vi "Setup.vi"() -> ()   [LabVIEW 2021, in "Main.lvlib"]
doc: "This VI is used to SetUP the signal properties. \n1.Start SetUP to view the signal\n2. Save Values to save the values that you pick to signal_values FGV\n3. Stop SetUP to stop the SetUP\n5. Exit SetUp"
uses:
  Main.lvlib
  Tipski Definicii/Setup_sostojbi.ctl
  Tipski Definicii/Signal Values.ctl
  Tipski Definicii/Unit.ctl
  Polymorphic/Init_SetUP.vi
  Polymorphic/DeQ_SetUP_QMH.vi
  Polymorphic/Enq_SetUP_QMH.vi
  Polymorphic/Release_SetUP.vi
  Signal/Signal.lvlib
  <vilib>/measure/NI_MABase.lvlib
  subVIS/Main_Programs_SubVIs.lvlib
  Polymorphic/Queues.lvlib
panel:
  in  "Stop SetUP":bool
  in  "Waveform":T1(ring)
  in  "Phase":dbl
  in  "Offset":dbl
  in  "Hz Value":dbl=10000.0 min=-10000.0 max=10000.0 step=0.001 format="%#.3f"
  in  "Amplitude":dbl min=-10.0 max=10.0 step=0.001 format="%#.3f"
  in  "Exit Setup":bool
  in  "Save Values":bool
  in  "Start Setup":bool
  out "Signal":waveform(dbl)(graph)
  # "For DC signal the waveform needs to be square. If you want to pick other waveform first change the f F"
  # "Waveform graph tools"
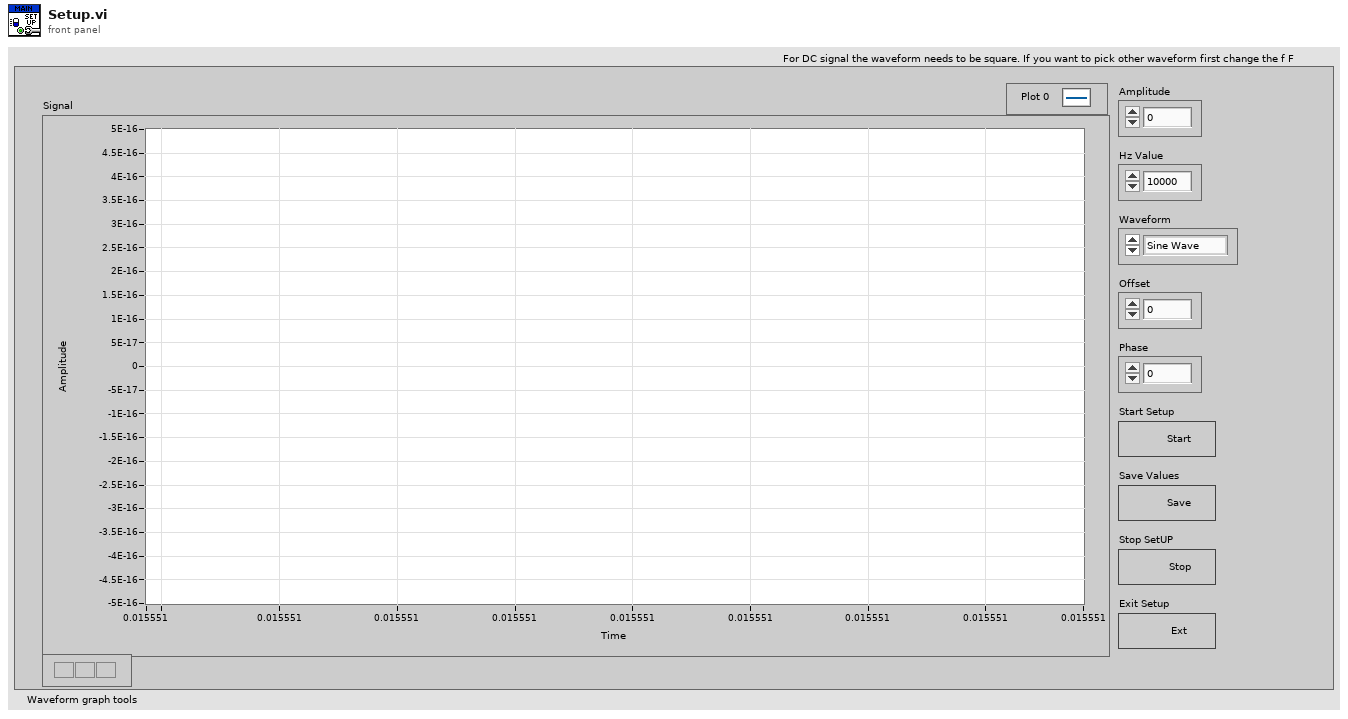
[diagram p1: front panel]
types:
  T1 = enum16{"Sine Wave", "Triangle Wave", "Square Wave", "Sawtooth Wave"}
  T2 = cluster{"Main Queue":refnum<queue>, "ER Refnum":refnum<event-registration>, "User Event":refnum<user-event>}
  T3 = typedef "SetUP_program_queues.ctl" = cluster{"Main Queue":refnum<queue>, "ER Refnum":refnum<event-registration>, "User Event":refnum<user-event>}
  T4 = typedef "Signal Values.ctl" = enum16{"Init", "Add V/A string", "Add Hz string", "Get Strings and Values", "Reset", "Add Offset", "Add Waveform", "Add Phase"}
  T5 = typedef "Setup_sostojbi.ctl" = enum16{"Init", "Generate Message ", "Setup", "End"}
  T6 = enum32{"Invalid", "Standard", "Closed", "Hidden", "Minimized", "Maximized"}
  T7 = cluster{"Amp String":string, "Amp Value":dbl, "Hz Value Out":dbl, "Waveform Out":enum16{"Sine Wave", "Triangle Wave", "Square Wave", "Sawtooth Wave"}, "Offset Out":dbl, "Phase Out":dbl, "Signal String":string, "Signal":waveform(dbl)}
  T8 = typedef "Unit.ctl" = enum16{"Init", "Add", "Read"}
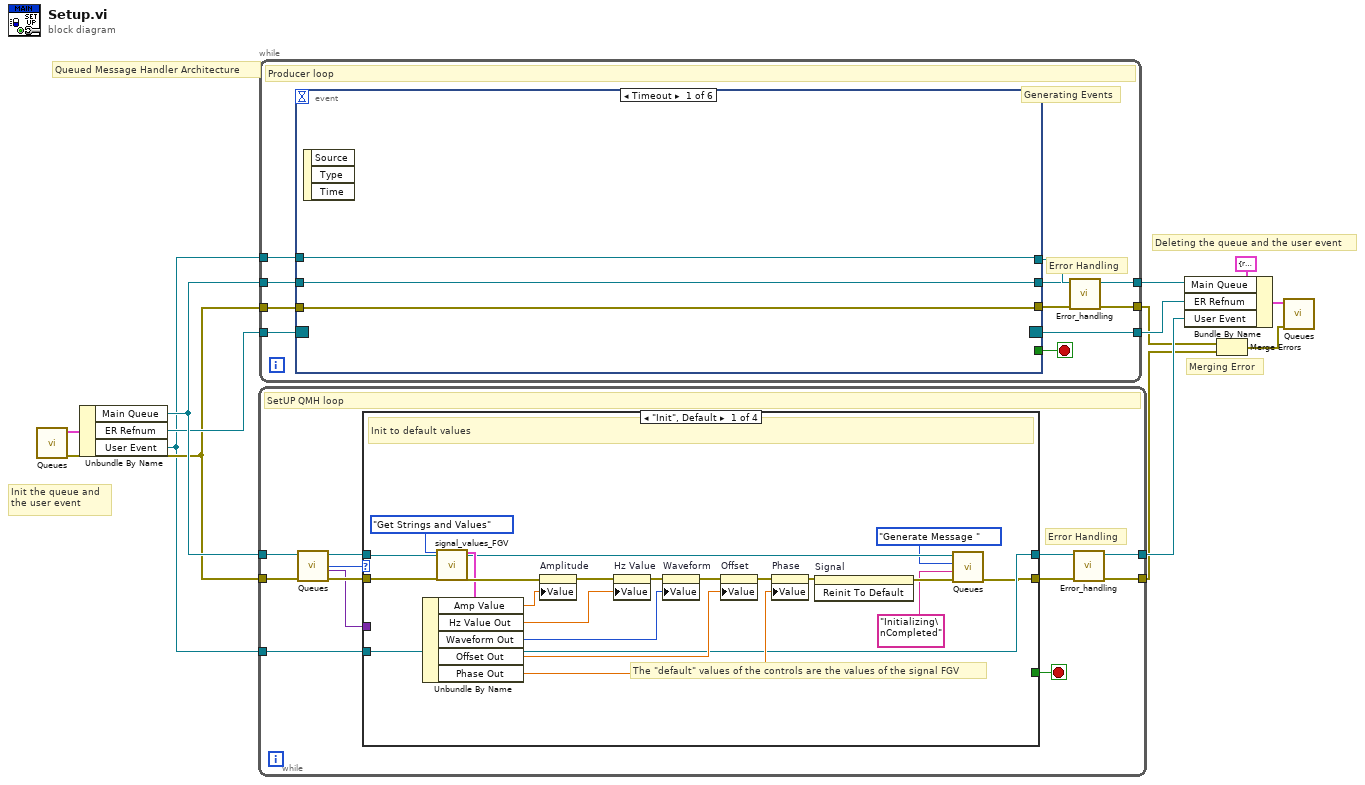
[diagram p0: block diagram]
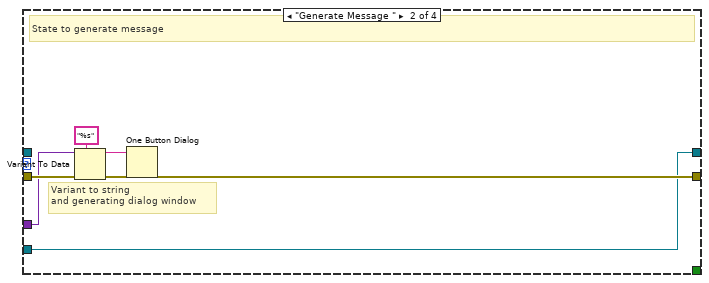
[diagram p2: hidden frame]
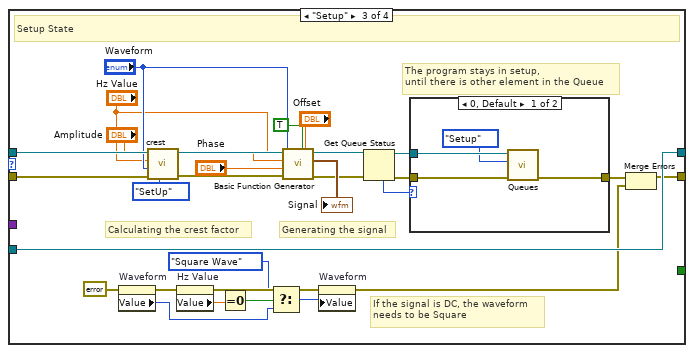
[diagram p3: hidden frame]
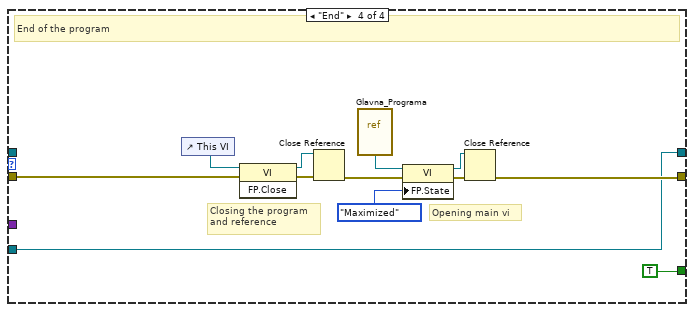
[diagram p5: hidden frame]
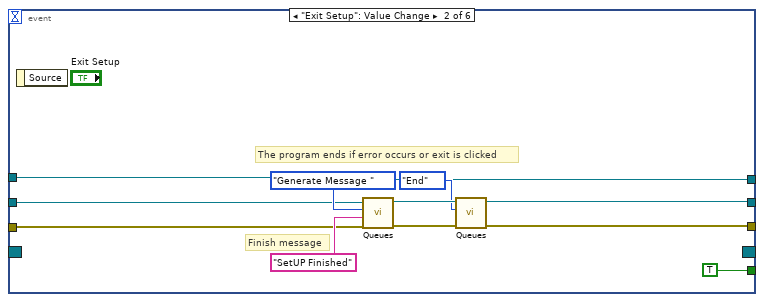
[diagram p6: hidden frame]
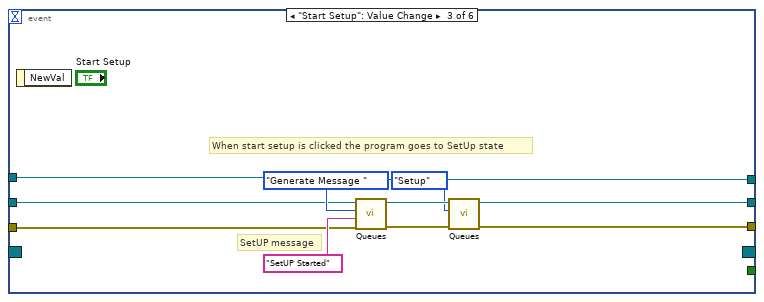
[diagram p7: hidden frame]
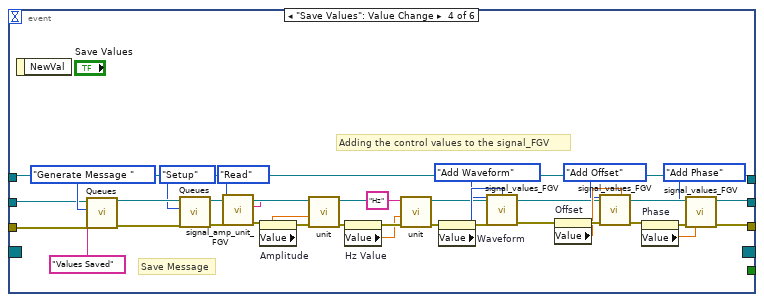
[diagram p8: hidden frame]
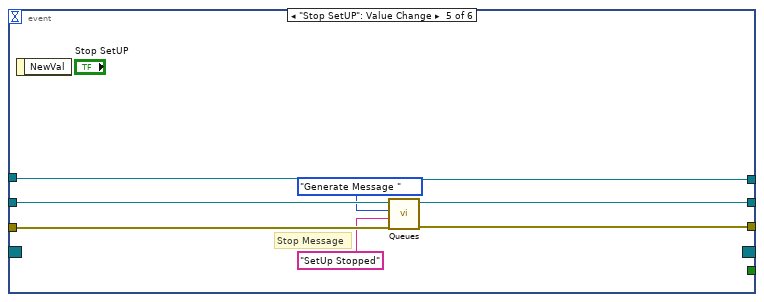
[diagram p9: hidden frame]
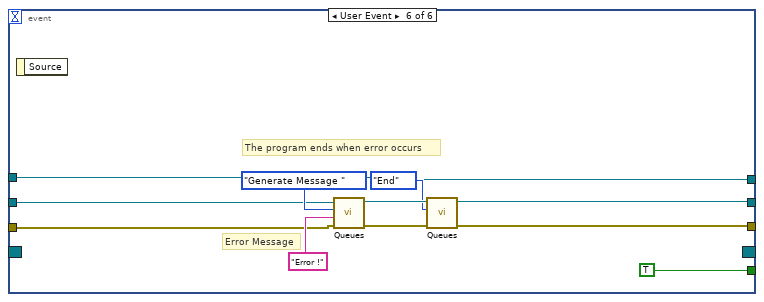
[diagram p10: hidden frame]
diagram:
  # "Merging Error"
  # "Deleting the queue and the user event"
  # "Init the queue and \nthe user event"
  # "Queued Message Handler Architecture"
  n1 = call-poly "Queues.vi"() -> ("Error Out"=w11:errorcluster, "Queue Cluster"=w10:T3)  [unwired: 10 in]
  n2 = Unbundle By Name(w10) -> ("Main Queue"=w13:refnum<queue>, "ER Refnum"=w12:refnum<event-registration>, "User Event"=w9:refnum<user-event>)
  n3 = while {
    tunnel: w13 -> [w18]
    tunnel: [w22] -> w5
    tunnel: w11 -> [w17]
    tunnel: [w24] -> w3
    tunnel: w9 -> [w21]
    stop <- w25 stop-if-true
    # "Error Handling"
    # "SetUP QMH loop"
    n4 = call-poly "Queues.vi"("Error In"=w17, "Queue In"=w18) -> ("Error Out"=w16:errorcluster, "Message"=w14:variant, "Instruction"=w15:T5, "Queue Out"=w19:refnum<queue>)  [unwired: 6 in]
    n5 = case shown="\"Init\", Default" w15 {
      tunnel: w19 -> [w30 _ w71 _]
      tunnel: [w31 w47 w56 w86] -> w23
      tunnel: [_ _ _ TRUE] -> w25
      tunnel: w16 -> [w39 w51 w68 w94]
      tunnel: w14 -> [_ w50 _ _]
      tunnel: w21 -> [w33 w46 w69 w85]
      tunnel: [w33 w46 w69 w85] -> w20
      frame "Init", Default {
        # "The \"default\" values of the controls are the values of the signal FGV"
        # "Init to default values"
        n6 = call "signal_values_FGV.vi"("Action"=Signal_Values."Get Strings and Values", "Error In"=w39) -> ("Signal"=w38:T7, "Error Out"=w45:errorcluster)  [unwired: 12 in]
        n7 = Unbundle By Name(w38) -> ("Amp Value"=w37:dbl, "Hz Value Out"=w36:dbl, "Waveform Out"=w27:T1, "Offset Out"=w35:dbl, "Phase Out"=w34:dbl)
        n8 = property on="Amplitude" class="DigNum (strict)"(error in=w45, "Value"=w37) -> (error out=w44:errorcluster)  [unwired: 1 in, 1 out]
        n9 = property on="Hz Value" class="DigNum (strict)"(error in=w44, "Value"=w36) -> (error out=w43:errorcluster)  [unwired: 1 in, 1 out]
        n10 = property on="Waveform" class="Enum (strict)"(error in=w43, "Value"=w27) -> (error out=w42:errorcluster)  [unwired: 1 in, 1 out]
        n11 = property on="Offset" class="DigNum (strict)"(error in=w42, "Value"=w35) -> (error out=w41:errorcluster)  [unwired: 1 in, 1 out]
        n12 = property on="Phase" class="DigNum (strict)"(error in=w41, "Value"=w34) -> (error out=w40:errorcluster)  [unwired: 1 in, 1 out]
        n13 = invoke on="Signal" class="WFGraph (strict)" method="Reinit To Default"(error in=w40) -> (error out=w32:errorcluster)  [unwired: 2 in, 2 out]
        n14 = call-poly "Queues.vi"("Error In"=w32, "Message"="Initializing\nCompleted", "Instruction"=Setup_sostojbi."Generate Message ", "Queue Out"=w30) -> ("Error Out"=w31:errorcluster)  [unwired: 6 in, 1 out]
      }
      frame "Generate Message " {
        # "Variant to string\nand generating dialog window"
        # "State to generate message"
        n15 = Variant To Data(error in=w51, type="%s", Variant=w50) -> (data=w48:string, error out=w47:errorcluster)
        n16 = One Button Dialog(message=w48) -> ()  [unwired: 1 in, 1 out]
      }
      frame "Setup" {
        # "Calculating the crest factor"
        # "If the signal is DC, the waveform\nneeds to be Square"
        # "The program stays in setup,\nuntil there is other element in the Queue"
        # "Generating the signal"
        # "Setup State"
        n17 = property on="Waveform" class="Enum (strict)"(error in=errorcluster {"status"=FALSE, "code"=0, "source"=""} ("error in (no error)")) -> (error out=w60:errorcluster, "Value"=w59:T1)  [unwired: 1 in, 1 out]
        n18 = call "crest.vi"("Set / Unit?"=enum16{"Unit", "SetUp"}."SetUp", "Error In"=w68, "SetUP W"="Waveform", "SetUP F"="Hz Value", "RMS"="Amplitude") -> ("Error Out"=w67:errorcluster, "Max"=w65:dbl)  [unwired: 5 in]
        n19 = property on="Hz Value" class="DigNum (strict)"(error in=w60) -> (error out=w79:errorcluster, "Value"=w64:dbl)  [unwired: 1 in, 1 out]
        n20 = Equal To 0?(x=w64) -> (x = 0?=w63:bool)
        n21 = Select(t=T1."Square Wave" ("Waveform"), s=w63, f=w59) -> (s? t:f=w58:T1)
        n22 = call <vilib>:"Basic Function Generator.vi"("offset"="Offset", "reset signal"=TRUE, "signal type"="Waveform", "error in (no error)"=w67, "phase"="Phase", "amplitude"=w65, "frequency"="Hz Value") -> ("error out"=w72:errorcluster, "signal out"=→"Signal":waveform(dbl))  [unwired: 2 in, 1 out]
        n23 = property on="Waveform" class="Enum (strict)"(error in=w79, "Value"=w58) -> (error out=w55:errorcluster)  [unwired: 1 in, 1 out]
        n24 = Get Queue Status(queue=w71, error in (no error)=w72) -> (queue out=w74:refnum<queue>, error out=w73:errorcluster, # elements in queue=w75:i32)  [unwired: 1 in, 5 out]
        n25 = case shown="0, Default" w75 {
          tunnel: w74 -> [w82 _]
          tunnel: w73 -> [w83 w84]
          tunnel: [w80 w84] -> w57
          frame 0, Default {
            n26 = call-poly "Queues.vi"("Error In"=w83, "Instruction"=Setup_sostojbi."Setup", "Queue Out"=w82) -> ("Error Out"=w80:errorcluster)  [unwired: 7 in, 1 out]
          }
          frame 1 {
          }
        }
        n27 = Merge Errors(w57, w55) -> (w56:errorcluster)
      }
      frame "End" {
        # "Opening main vi"
        # "Closing the program\nand reference"
        # "End of the program"
        n28 = control-ref of="This VI"() -> (w95:refnum<vi>)
        n29 = invoke class="VI" method="FP.Close"(reference=w95, error in=w94) -> (reference out=w92:refnum<vi>, error out=w93:errorcluster)  [unwired: 1 in, 1 out]
        n30 = Close Reference(reference=w92, error in (no error)=w93) -> (error out=w91:errorcluster)
        n31 = vi-ref "Glavna_Programa.vi"() -> (w90:refnum<vi>)
        n32 = property class="VI"(reference=w90, error in=w91, "FP.State"=T6."Maximized" ("Front Panel Window:State")) -> (reference out=w87:refnum<vi>, error out=w88:errorcluster)
        n33 = Close Reference(reference=w87, error in (no error)=w88) -> (error out=w86:errorcluster)
      }
    }
    n34 = call "Error_handling.vi"("Error In"=w23, "User Event in"=w20) -> ("Error Out"=w24:errorcluster, "User Event out"=w22:refnum<user-event>)  [unwired: 8 in]
  }
  n35 = while {
    tunnel: w11 -> [w105]
    tunnel: w13 -> [w106]
    tunnel: w12 -> [w104]
    tunnel: [w103] -> w6
    tunnel: w9 -> [w101]
    tunnel: [w99] -> w7
    tunnel: [w98] -> w4
    stop <- w97 stop-if-true
    # "Error Handling"
    # "Generating Events"
    # "Producer loop"
    n36 = event shown="[0] Timeout" {
      selector: w104 -> [_ _ _ _ _ _]
      dyn-events: [_ _ _ _ _ _] -> w103
      timeout: _ -> [_ _ _ _ _ _]
      tunnel: w106 -> [w109 w113 w124 w143 w166 w173]
      tunnel: [w109 w112 w121 w139 w167 w172] -> w99
      tunnel: w105 -> [w108 w114 w125 w144 w169 w174]
      tunnel: [w108 w111 w122 w147 w168 w171] -> w102
      tunnel: [_ TRUE _ _ _ TRUE] -> w97
      tunnel: w101 -> [w107 w110 w123 w142 w163 w170]
      tunnel: [w107 w110 w123 w142 w163 w170] -> w100
      event Timeout {
        n37 = event-data() -> ()  [unwired: 1 in, 3 out]
      }
      event "Exit Setup": Value Change {
        # "Finish message"
        # "The program ends if error occurs or exit is clicked"
        n38 = event-data() -> ()  [unwired: 1 in, 1 out]
        n39 = call-poly "Queues.vi"("Error In"=w114, "Message"="SetUP Finished", "Instruction"=Setup_sostojbi."Generate Message ", "Queue Out"=w113) -> ("Error Out"=w118:errorcluster, "Queue Out"=w119:refnum<queue>)  [unwired: 6 in]
        n40 = call-poly "Queues.vi"("Error In"=w118, "Instruction"=Setup_sostojbi."End", "Queue Out"=w119) -> ("Error Out"=w111:errorcluster, "Queue Out"=w112:refnum<queue>)  [unwired: 7 in]
      }
      event "Start Setup": Value Change {
        # "SetUP message"
        # "When start setup is clicked the program goes to SetUp state"
        n41 = event-data() -> ()  [unwired: 1 in, 1 out]
        n42 = call-poly "Queues.vi"("Error In"=w125, "Message"="SetUP Started", "Instruction"=Setup_sostojbi."Generate Message ", "Queue Out"=w124) -> ("Error Out"=w129:errorcluster, "Queue Out"=w130:refnum<queue>)  [unwired: 6 in]
        n43 = call-poly "Queues.vi"("Error In"=w129, "Instruction"=Setup_sostojbi."Setup", "Queue Out"=w130) -> ("Error Out"=w122:errorcluster, "Queue Out"=w121:refnum<queue>)  [unwired: 7 in]
      }
      event "Save Values": Value Change {
        # "Save Message"
        # "Adding the control values to the signal_FGV"
        n44 = event-data() -> ()  [unwired: 1 in, 1 out]
        n45 = call-poly "Queues.vi"("Error In"=w144, "Message"="Values Saved", "Instruction"=Setup_sostojbi."Generate Message ", "Queue Out"=w143) -> ("Error Out"=w141:errorcluster, "Queue Out"=w140:refnum<queue>)  [unwired: 6 in]
        n46 = call-poly "Queues.vi"("Error In"=w141, "Instruction"=Setup_sostojbi."Setup", "Queue Out"=w140) -> ("Error Out"=w134:errorcluster, "Queue Out"=w139:refnum<queue>)  [unwired: 7 in]
        n47 = call "signal_amp_unit_FGV.vi"("Error In"=w134, "Action"=Unit."Read") -> ("Error Out"=w133:errorcluster, "Base"=w131:string)  [unwired: 7 in, 1 out]
        n48 = property on="Amplitude" class="DigNum (strict)"(error in=w133) -> (error out=w162:errorcluster, "Value"=w161:dbl)  [unwired: 1 in, 1 out]
        n49 = call "unit.vi"("Error In"=w162, "Signal Amp"=w161, "Unit"=w131) -> ("Error Out"=w160:errorcluster)  [unwired: 8 in]
        n50 = property on="Hz Value" class="DigNum (strict)"(error in=w160) -> (error out=w159:errorcluster, "Value"=w158:dbl)  [unwired: 1 in, 1 out]
        n51 = call "unit.vi"("Error In"=w159, "Signal Amp"=w158, "Unit"="Hz") -> ("Error Out"=w156:errorcluster)  [unwired: 8 in]
        n52 = property on="Waveform" class="Enum (strict)"(error in=w156) -> (error out=w154:errorcluster, "Value"=w155:T1)  [unwired: 1 in, 1 out]
        n53 = call "signal_values_FGV.vi"("Action"=Signal_Values."Add Waveform", "Waveform"=w155, "Error In"=w154) -> ("Error Out"=w153:errorcluster)  [unwired: 11 in, 1 out]
        n54 = property on="Offset" class="DigNum (strict)"(error in=w153) -> (error out=w152:errorcluster, "Value"=w151:dbl)  [unwired: 1 in, 1 out]
        n55 = call "signal_values_FGV.vi"("Action"=Signal_Values."Add Offset", "Offset"=w151, "Error In"=w152) -> ("Error Out"=w150:errorcluster)  [unwired: 11 in, 1 out]
        n56 = property on="Phase" class="DigNum (strict)"(error in=w150) -> (error out=w149:errorcluster, "Value"=w148:dbl)  [unwired: 1 in, 1 out]
        n57 = call "signal_values_FGV.vi"("Action"=Signal_Values."Add Phase", "Error In"=w149, "Phase"=w148) -> ("Error Out"=w147:errorcluster)  [unwired: 11 in, 1 out]
      }
      event "Stop SetUP": Value Change {
        # "Stop Message"
        n58 = event-data() -> ()  [unwired: 1 in, 1 out]
        n59 = call-poly "Queues.vi"("Error In"=w169, "Message"="SetUp Stopped", "Instruction"=Setup_sostojbi."Generate Message ", "Queue Out"=w166) -> ("Error Out"=w168:errorcluster, "Queue Out"=w167:refnum<queue>)  [unwired: 6 in]
      }
      event User Event {
        # "The program ends when error occurs"
        # "Error Message"
        n60 = event-data() -> ()  [unwired: 1 in, 1 out]
        n61 = call-poly "Queues.vi"("Error In"=w174, "Message"="Error !", "Instruction"=Setup_sostojbi."Generate Message ", "Queue Out"=w173) -> ("Error Out"=w178:errorcluster, "Queue Out"=w179:refnum<queue>)  [unwired: 6 in]
        n62 = call-poly "Queues.vi"("Error In"=w178, "Instruction"=Setup_sostojbi."End", "Queue Out"=w179) -> ("Error Out"=w171:errorcluster, "Queue Out"=w172:refnum<queue>)  [unwired: 7 in]
      }
    }
    n63 = call "Error_handling.vi"("Error In"=w102, "User Event in"=w100) -> ("Error Out"=w98:errorcluster)  [unwired: 8 in, 1 out]
  }
  n64 = Bundle By Name(cluster=T2 {"Main Queue"=refnum, "ER Refnum"=refnum, "User Event"=refnum} ("Queue Cluster"), "Main Queue"=w7, "ER Refnum"=w6, "User Event"=w5) -> (w1:T2)
  n65 = Merge Errors(w4, w3) -> (w2:errorcluster)
  n66 = call-poly "Queues.vi"("Error In"=w2, "Queue Cluster"=w1) -> ()  [unwired: 10 in]
